vi "Create.vi"(8 "error in (no error)":errorcluster, 10 "TreeControl in":refnum<vi>) -> (0 "error out":errorcluster, 3 "Tag Tree out":refnum<class "Tag Tree.lvclass">)   [LabVIEW 2020, in "Tag Tree.lvclass"]
uses:
  Tag Tree.lvclass
  Tag Tree.lvclass/Tag Tree.ctl
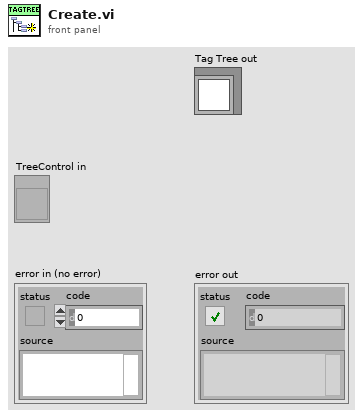
[diagram p1: front panel]
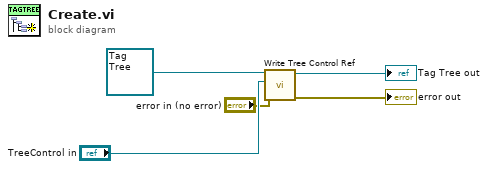
[diagram p0: block diagram]
diagram:
  n1 = call "Write Tree Control Ref.vi"("error in (no error)"="error in (no error)", "Tag Tree Reference"="TreeControl in", "Tag Tree In"=refnum<class "Tag Tree.lvclass"> refnum ("Support Utilities.lvlib:Tag Tree.lvclass")) -> ("error out"=→"error out":errorcluster, "Tag Tree Out"=→"Tag Tree out":refnum<class "Tag Tree.lvclass">)  [unwired: 7 in]
